vi "System@WarningBox__Parameter.vi"(1 "ParamterIn":string) -> (0 "ParamterOut":string)   [LabVIEW 2020]
panel:
  in  "LogMessage":string(combo)
  in  "UserMessage":string(combo)
  in  "Logic":string(combo)
  in  "Confirm":bool
  # "System@WarningBox $Logic,$UserMessage(,$LogMessage)"
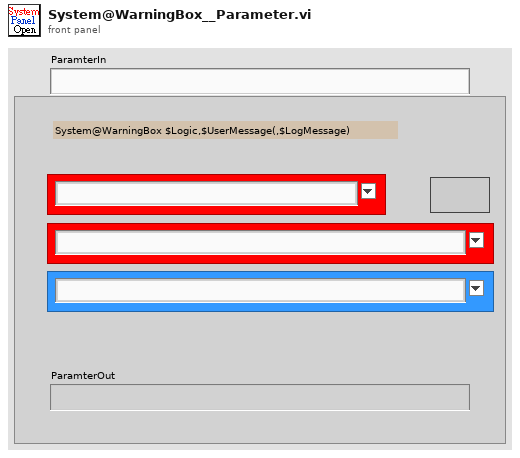
[diagram p1: front panel]
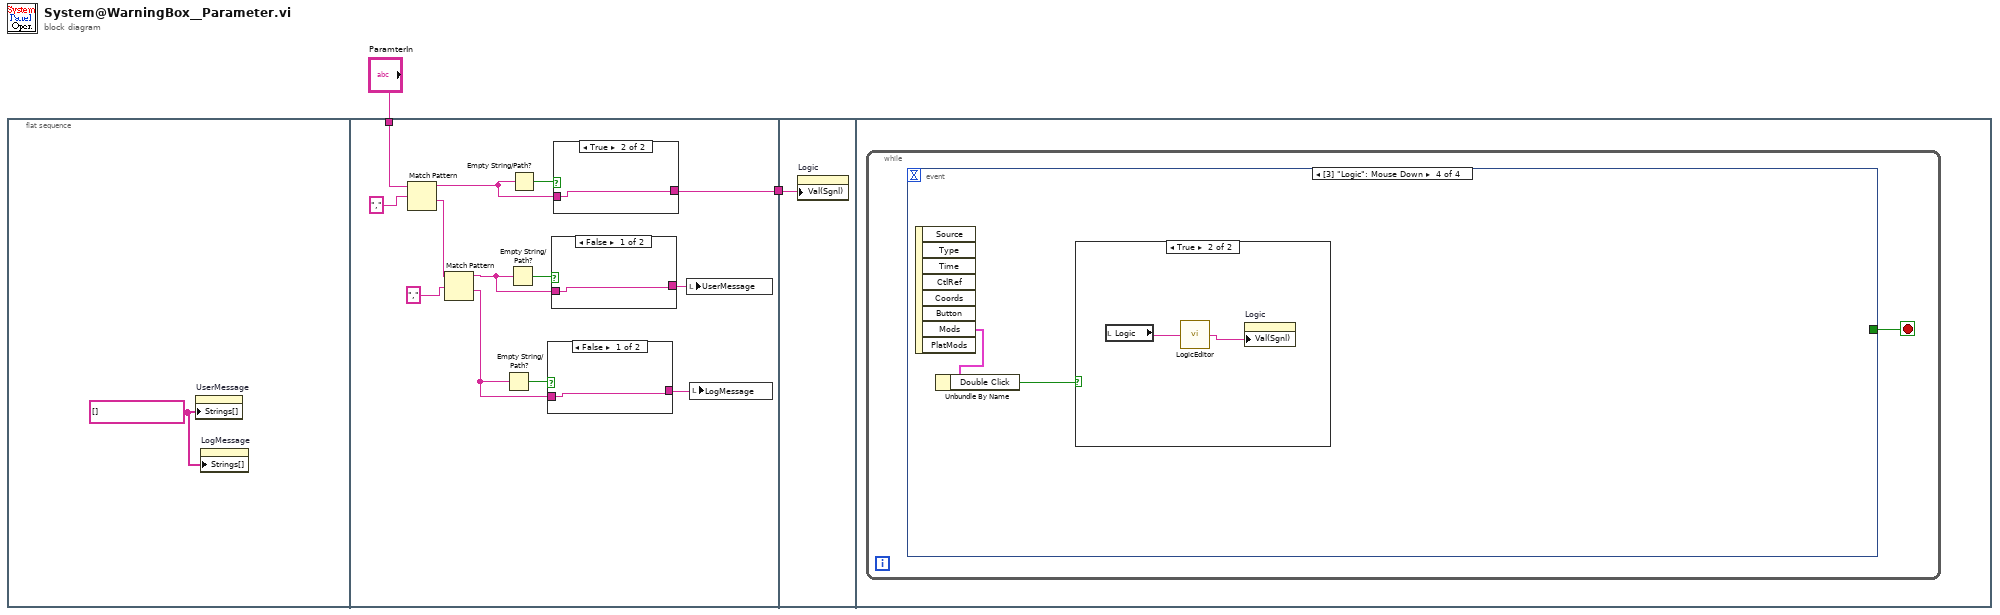
[diagram p0: block diagram]
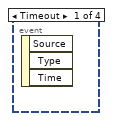
[diagram p5: hidden frame]
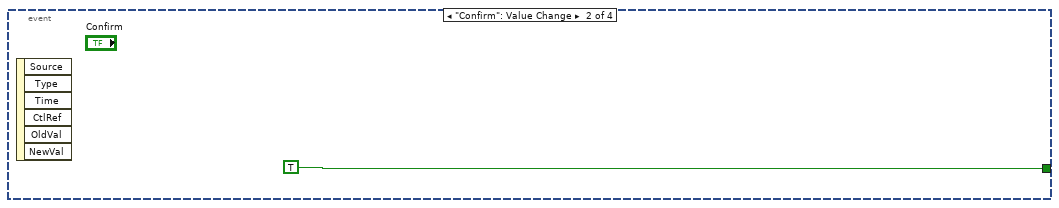
[diagram p6: hidden frame]
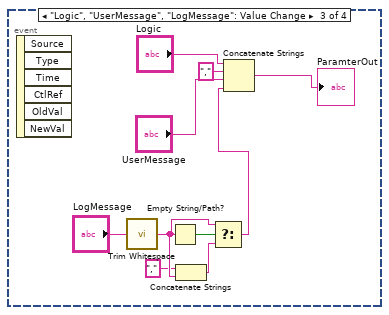
[diagram p7: hidden frame]
diagram:
  n1 = flat-sequence {
    tunnel: "ParamterIn" -> [w15]
    tunnel: [w11] -> w1
    tunnel: w1 -> [w23]
    frame #0 {
      w3 = string[] [] ("Strings []")
      n2 = property on="UserMessage" class="CmbBox"("Strings[]"=w3) -> ()  [unwired: 2 in, 2 out]
      n3 = property on="LogMessage" class="CmbBox"("Strings[]"=w3) -> ()  [unwired: 2 in, 2 out]
    }
    frame #1 {
      n4 = Match Pattern(string=w15, regular expression=",") -> (before substring=w13:string, after substring=w8:string)  [unwired: 1 in, 2 out]
      n5 = Match Pattern(string=w8, regular expression=",") -> (before substring=w7:string, after substring=w5:string)  [unwired: 1 in, 2 out]
      n6 = Empty String/Path?(string/path=w5) -> (empty?=w6:bool)
      n7 = Empty String/Path?(string/path=w7) -> (empty?=w12:bool)
      n8 = Empty String/Path?(string/path=w13) -> (empty?=w16:bool)
      n9 = case shown="False" w6 {
        tunnel: w5 -> [w17 w18]
        tunnel: [w17 w18] -> w4
        frame False {
        }
        frame True {
        }
      }
      n10 = case shown="False" w12 {
        tunnel: w7 -> [w19 w20]
        tunnel: [w19 w20] -> w10
        frame False {
        }
        frame True {
        }
      }
      n11 = case shown="True" w16 {
        tunnel: w13 -> [w21 w22]
        tunnel: [w21 w22] -> w11
        frame False {
        }
        frame True {
        }
      }
      n12 = local write "UserMessage"(w10) -> ()
      n13 = local write "LogMessage"(w4) -> ()
    }
    frame #2 {
      n14 = property on="Logic" class="CmbBox"("Val(Sgnl)"=w23) -> ()  [unwired: 2 in, 2 out]
    }
    frame #3 {
      n15 = while {
        stop <- w24 stop-if-true
        n16 = event shown="[3] \"Logic\": Mouse Down" {
          selector: _ -> [_ _ _ _]
          dyn-events: _ -> [_ _ _ _]
          timeout: _ -> [_ _ _ _]
          tunnel: [_ TRUE _ _] -> w24
          event Timeout {
            n17 = event-data() -> ()  [unwired: 1 in, 3 out]
          }
          event "Confirm": Value Change {
            n18 = event-data() -> ()  [unwired: 1 in, 6 out]
          }
          event "Logic", "UserMessage", "LogMessage": Value Change {
            n19 = event-data() -> ()  [unwired: 1 in, 6 out]
            n20 = call <vilib>:"Trim Whitespace.vi"("string"="LogMessage") -> ("trimmed string"=w29:string)  [unwired: 1 in]
            n21 = Empty String/Path?(string/path=w29) -> (empty?=w30:bool)
            n22 = Concatenate Strings("," ("string"), w29) -> (w27:string)
            n23 = Select(t=w29, s=w30, f=w27) -> (s? t:f=w26:string)
            n24 = Concatenate Strings("Logic", "," ("string"), "UserMessage", w26) -> (→"ParamterOut":string)
          }
          event "Logic": Mouse Down {
            n25 = event-data() -> ("Mods"=w37:cluster{"Double Click":bool, "Menu Key":bool})  [unwired: 1 in, 7 out]
            n26 = Unbundle By Name(w37) -> ("Double Click"=w36:bool)
            n27 = case shown="True" w36 {
              frame False {
              }
              frame True {
                n28 = local read "Logic"() -> (w39:string)
                n29 = call "LogicEditor.vi"("Logic Express"=w39) -> ("LogicExpressOut"=w38:string)
                n30 = property on="Logic" class="CmbBox"("Val(Sgnl)"=w38) -> ()  [unwired: 2 in, 2 out]
              }
            }
          }
        }
      }
    }
  }
